vi "Update UI Project.vi"(8 "error in (no error)":errorcluster, 10 "New Name":string, 11 "Template Project Path":path) -> (0 "error out":errorcluster)   [LabVIEW 2021, in "Plugin Generator.lvlib"]
uses:
  Plugin Generator.lvlib
  Scripting Utilities/LV Scripting Utilities.lvlib
  <vilib>/Utility/EditLVProj/Edit LVProj.lvlib
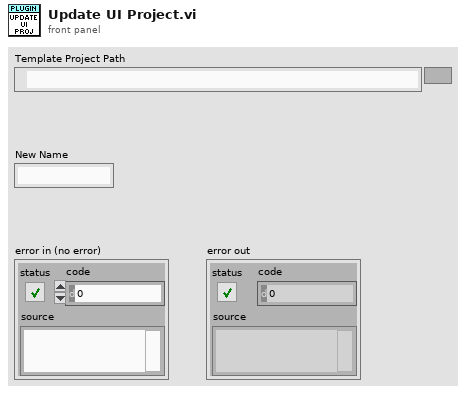
[diagram p1: front panel]
types:
  T1 = cluster{"Library Name":string, "Update Folder Name":bool}[]
  T2 = typedef "Edit LVProj.lvlib/Library And VI References.ctl" = cluster{"Target Reference":refnum<vi>, "VI References":refnum<vi>[], "Library References":refnum<vi>[]}
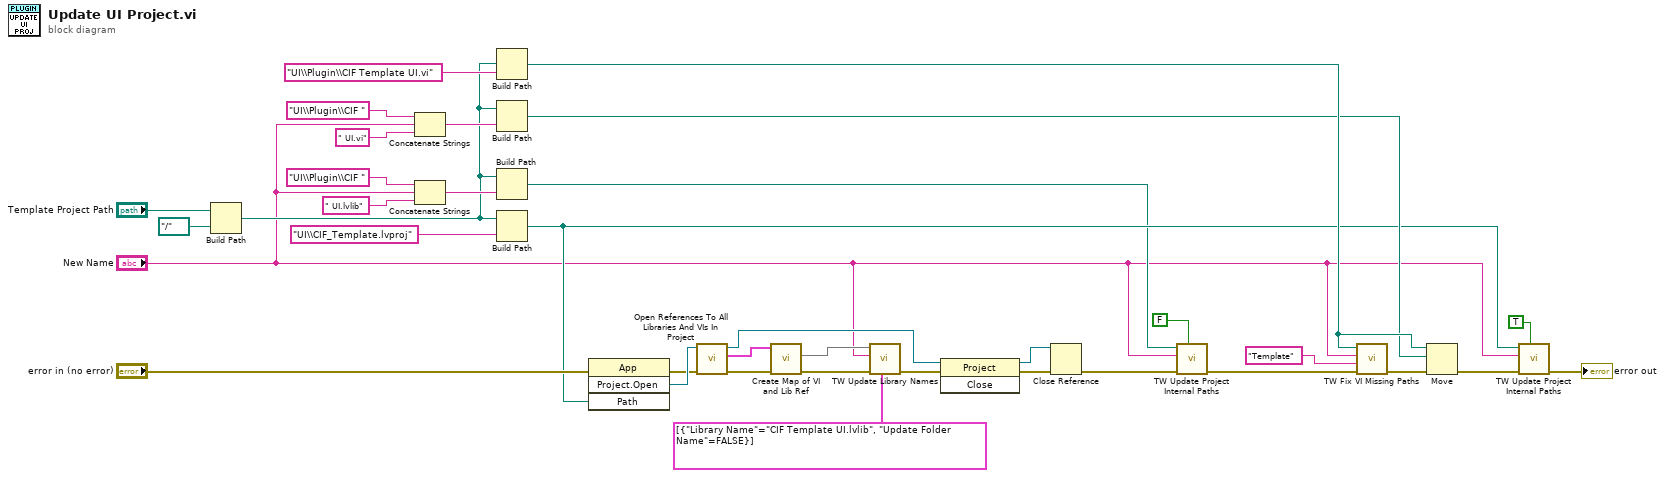
[diagram p0: block diagram]
diagram:
  n1 = Build Path(base path="Template Project Path", name or relative path=path "../..") -> (appended path=w3:path)
  n2 = Concatenate Strings("UI\\Plugin\\CIF " ("Class Name"), "New Name", " UI.vi" ("Class Name")) -> (w26:string)
  n3 = Concatenate Strings("UI\\Plugin\\CIF " ("Class Name"), "New Name", " UI.lvlib" ("Class Name")) -> (w4:string)
  n4 = Build Path(base path=w3, name or relative path="UI\\Plugin\\CIF Template UI.vi" ("Class Name")) -> (appended path=w29:path)
  n5 = Build Path(base path=w3, name or relative path=w26) -> (appended path=w25:path)
  n6 = Build Path(base path=w3, name or relative path=w4) -> (appended path=w19:path)
  n7 = Build Path(base path=w3, name or relative path="UI\\CIF_Template.lvproj" ("Class Name")) -> (appended path=w20:path)
  n8 = invoke class="App" method="Project.Open"(error in="error in (no error)", "Path"=w20) -> (error out=w14:errorcluster, "Project:Open"=w17:refnum<vi>)  [unwired: 2 in, 2 out]
  n9 = call <vilib>:"Open References To All Libraries And VIs In Project.vi"("error in (no error)"=w14, "Project in"=w17) -> ("error out"=w13:errorcluster, "VI and Library References"=w18:T2[], "Project out"=w9:refnum<vi>)  [unwired: 7 in]
  n10 = call "Create Map of VI and Lib Ref.vi"("error in"=w13, "VI and Library References"=w18) -> ("error out"=w10:errorcluster, "Library Map"=w11:map{string, refnum<vi>})  [unwired: 7 in, 1 out]
  n11 = call "TW Update Library Names.vi"("Libraries"=T1 [{"Library Name"="CIF Template UI.lvlib", "Update Folder Name"=FALSE}], "error in"=w10, "New Subname"="New Name", "Library Map"=w11) -> ("error out"=w8:errorcluster)  [unwired: 6 in, 1 out]
  n12 = invoke class="Project" method="Close"(reference=w9, error in=w8) -> (reference out=w15:refnum<vi>, error out=w16:errorcluster)  [unwired: 1 in, 1 out]
  n13 = Close Reference(reference=w15, error in (no error)=w16) -> (error out=w23:errorcluster)
  n14 = call "TW Update Project Internal Paths.vi"("Rename Project"=FALSE, "error in (no error)"=w23, "New Subname"="New Name", "Project Path"=w19) -> ("error out"=w22:errorcluster)  [unwired: 7 in]
  n15 = call "TW Fix VI Missing Paths.vi"("error in (no error)"=w22, "Replace Subname"="Template" ("Subname to Replace"), "New Subname"="New Name", "VI Path"=w29) -> ("error out"=w21:errorcluster)  [unwired: 7 in]
  n16 = Move(source path=w29, error in=w21, 10:w25) -> (error out=w24:errorcluster)  [unwired: 2 in, 2 out]
  n17 = call "TW Update Project Internal Paths.vi"("Rename Project"=TRUE, "error in (no error)"=w24, "New Subname"="New Name", "Project Path"=w20) -> ("error out"=→"error out":errorcluster)  [unwired: 7 in]
